vi "Close SubPanels.vi"(8 "Error In":errorcluster, 10 "Subpanel Ref (Block Diagram Preview)":refnum<vi>, 11 "Subpanel Ref (Front Panel Preview)":refnum<vi>) -> (0 "Error Out":errorcluster)   [LabVIEW 2022 SP3]
doc: "<add documentation here>"
panel:
  # "Development\nControls or indicators that are useful for development or testing, but which are not outputs of the VI."
  # "Input\nInputs to the VI"
  # "Output\nOutputs of the VI"
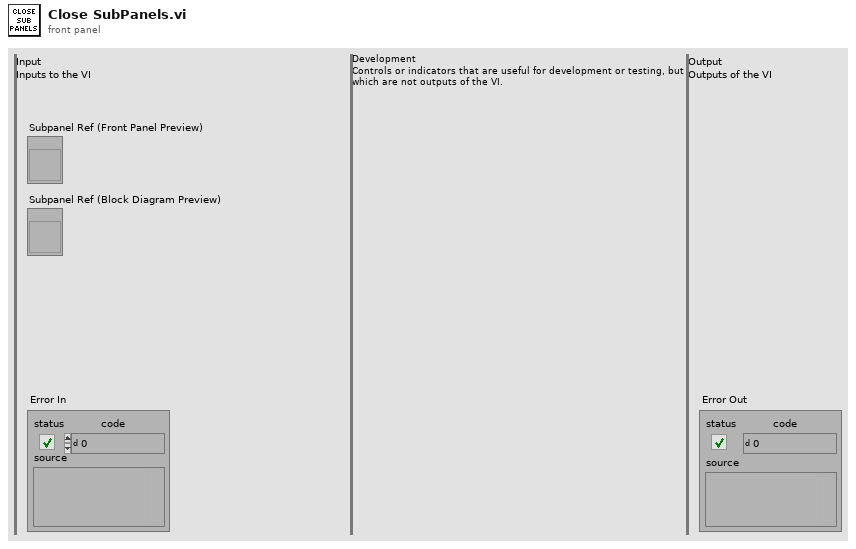
[diagram p1: front panel]
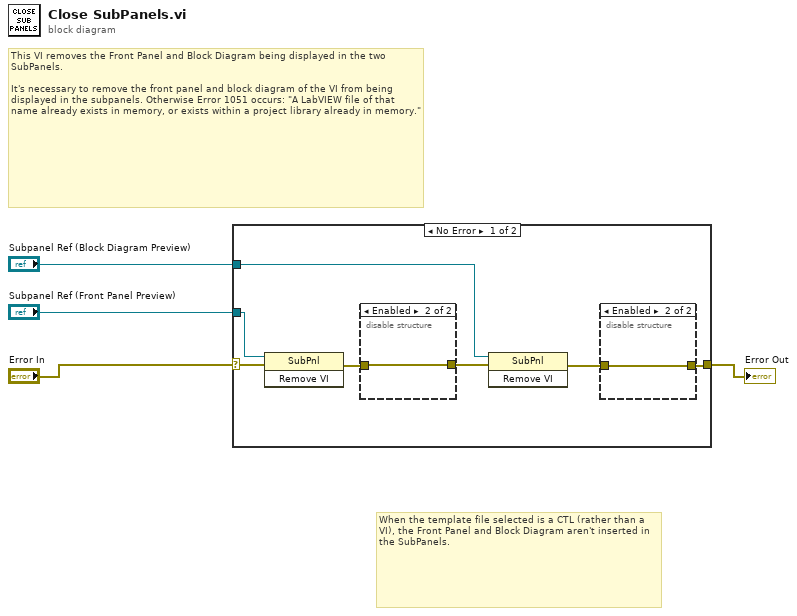
[diagram p0: block diagram]
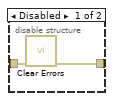
[diagram p2: hidden frame]
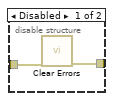
[diagram p3: hidden frame]
diagram:
  # "When the template file selected is a CTL (rather than a VI), the Front Panel and Block Diagram aren't inserted in the SubPanels."
  # "This VI removes the Front Panel and Block Diagram being displayed in the two SubPanels.\n\nIt's necessary to remove the front panel and block diagram of the VI from being displayed in the subpanels. Otherwise Error 1051 occurs: \"A LabVIEW file of that name already exists in memory, or exists within a project library already in memory.\""
  n1 = case shown="No Error" "Error In" {
    selector: "Error In" -> [w11 w18]
    tunnel: [w10 w18] -> w3
    tunnel: "Subpanel Ref (Front Panel Preview)" -> [w6 _]
    tunnel: "Subpanel Ref (Block Diagram Preview)" -> [w5 _]
    frame No Error {
      n2 = invoke on="Invoke Node" class="SubPnl" method="Remove VI"(reference=w6, error in=w11) -> (error out=w8:errorcluster)  [unwired: 1 in, 2 out]
      n3 = disable-structure shown="Enabled" {
        disable-tunnel: w8 -> [w16 w17]
        disable-tunnel: [w15 w17] -> w7
        frame Disabled {
          n4 = call <vilib>:"Clear Errors.vi"("error in (no error)"=w16) -> ("error out"=w15:errorcluster)  [unwired: 5 in, 1 out]
        }
        frame Enabled {
        }
      }
      n5 = invoke on="Invoke Node" class="SubPnl" method="Remove VI"(reference=w5, error in=w7) -> (error out=w9:errorcluster)  [unwired: 1 in, 2 out]
      n6 = disable-structure shown="Enabled" {
        disable-tunnel: [w13 w14] -> w10
        disable-tunnel: w9 -> [w12 w14]
        frame Disabled {
          n7 = call <vilib>:"Clear Errors.vi"("error in (no error)"=w12) -> ("error out"=w13:errorcluster)  [unwired: 5 in, 1 out]
        }
        frame Enabled {
        }
      }
    }
    frame Error {
    }
  }
  "Error Out" <- w3
